vi "Set ITC LPF Needle Valve.vi"(8 "error in (no error)":errorcluster, 10 "Percentage Open (%)":dbl format="%#.2f", 11 "Instrument.Oxford1820 in":refnum<class "Instrument.Oxford1820.lvclass">) -> (0 "error out":errorcluster, 2 "Response":string, 3 "Instrument.Oxford1820 out":refnum<class "Instrument.Oxford1820.lvclass">)   [LabVIEW 2016, in "Instrument.Oxford1820.lvclass"]
uses:
  Instrument.Oxford1820.lvclass
  Instrument.Oxford1820.lvclass/Instrument.Oxford1820.ctl
  <instrlib>/Mercury iXX/Public/Libraries/Lambda/Open/Open Lambda Device.vi
  <instrlib>/Mercury iXX/Public/Libraries/Lambda/Configuration/Set/Lambda Percentage Flow (Set).vi
  <instrlib>/Mercury iXX/Mercury iXX.lvlib
  <instrlib>/Mercury iXX/Public/Libraries/Lambda.lvlib
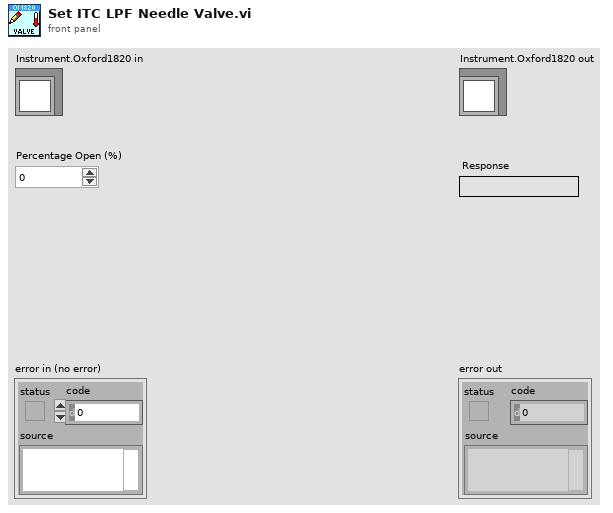
[diagram p1: front panel]
types:
  T1 = typedef "Mercury iXX.lvlib/Mercury Reference.ctl" = cluster{"Comms":refnum<visa-resource-name>, "Device ID":string[], "Comms Layer":T2, "Command":string, "Query reference":T3}
  T2 = typedef "Mercury iXX.lvlib/Comms Transport Layer.ctl" = enum16{"Ethernet TCP/IP", "USB", "ISOBus - RS-232", "GPIB"}
  T3 = typedef "Mercury iXX.lvlib/Query Dynamic Reference.ctl" = refnum<vi>
  T4 = typedef "Mercury iXX.lvlib/Response String.ctl" = string
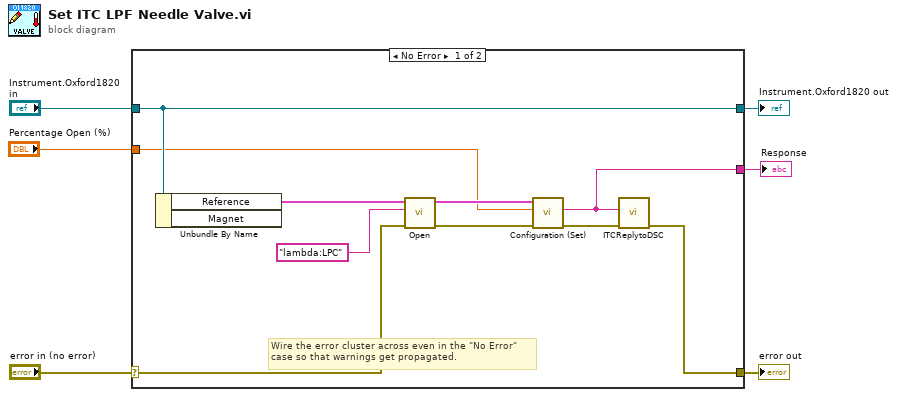
[diagram p0: block diagram]
diagram:
  n1 = case shown="No Error" "error in (no error)" {
    selector: "error in (no error)" -> [w13 w18]
    tunnel: [w8 w18] -> w5
    tunnel: [w16 w17] -> w3
    tunnel: "Instrument.Oxford1820 in" -> [w16 w17]
    tunnel: [w7 _] -> w2
    tunnel: "Percentage Open (%)" -> [w10 _]
    frame No Error {
      # "Wire the error cluster across even in the \"No Error\"\ncase so that warnings get propagated."
      n2 = Unbundle By Name(w16) -> ("Reference"=w14:T1)  [unwired: 1 out]
      n3 = call-poly <instrlib>:"Open.vi"("error in (no error)"=w13, "Device Identifier"="lambda:LPC", "Mercury Reference In"=w14) -> ("error out"=w12:errorcluster, "Mercury Reference Out"=w11:T1)  [unwired: 7 out]
      n4 = call-poly <instrlib>:"Configuration (Set).vi"("error in"=w12, "Percentage Open"=w10, "Mercury Reference In"=w11) -> ("error out"=w9:errorcluster, "Response"=w7:T4)  [unwired: 5 in, 2 out]
      n5 = call "ITCReplytoDSC.vi"("error in (no error)"=w9, "Response"=w7) -> ("error out"=w8:errorcluster)  [unwired: 9 in]
    }
    frame Error {
    }
  }
  "error out" <- w5
  "Instrument.Oxford1820 out" <- w3
  "Response" <- w2
